vi "core.vi"(8 "H[5] in":u32[](array[numeric]), 11 "W[80]":u32[](array[numeric])) -> (0 "H[5] out":u32[](array[numeric]))   [LabVIEW 2013, in "SHA-1.lvlib" / "SHA-1.lvclass"]
uses:
  SHA-1.lvclass
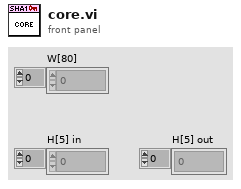
[diagram p1: front panel]
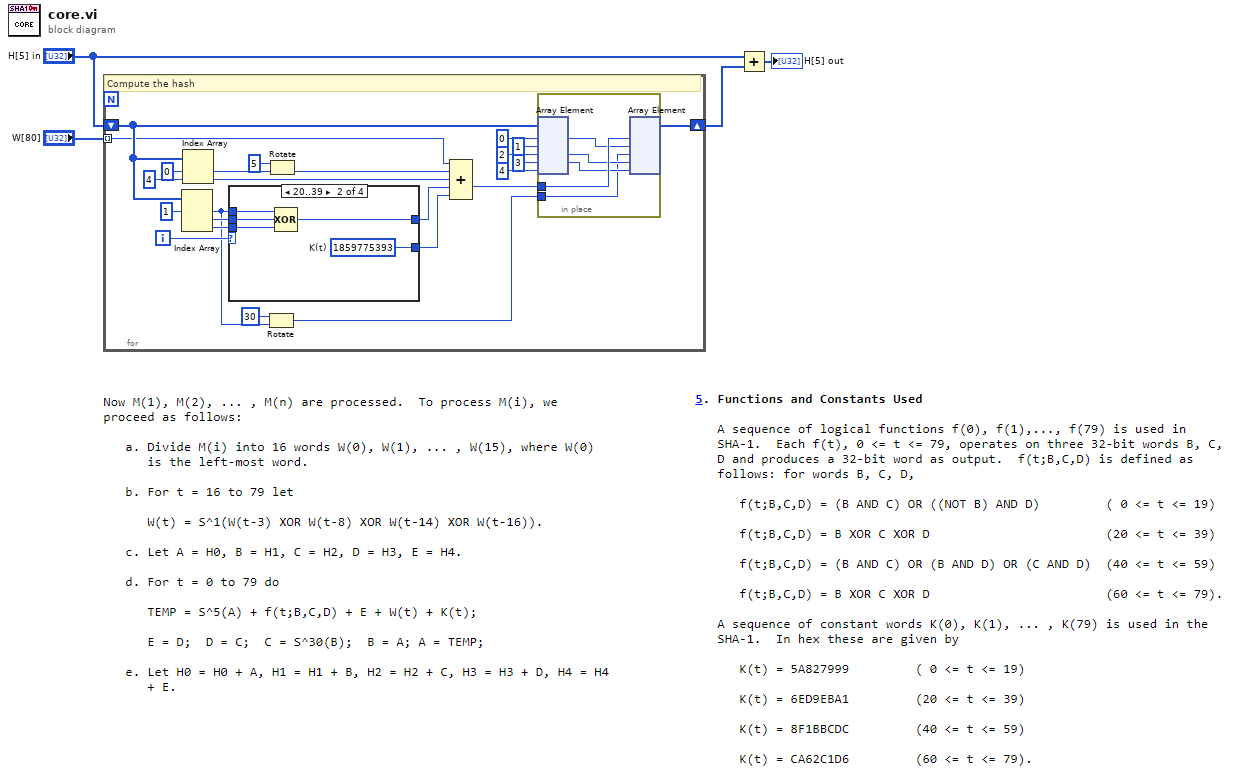
[diagram p0: block diagram]
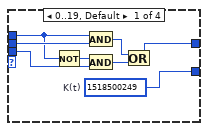
[diagram p2: hidden frame]
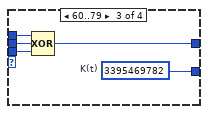
[diagram p3: hidden frame]
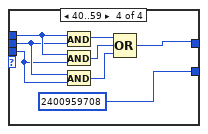
[diagram p4: hidden frame]
diagram:
  n1 = for {
    shift-right: [w9] -> w1
    shift-left: "H[5] in" -> [w18]
    tunnel: "W[80]" -> [w5] mode=indexing
    i -> [w28]
    # "Compute the hash"
    n2 = Index Array(array=w18, index #1=1 ("index")) -> (element #1=w16:u32, element #2=w21:u32, element #3=w20:u32)  [unwired: 2 in]
    n3 = Index Array(array=w18, index #1=0 ("index"), index #2=4 ("index")) -> (element #1=w24:u32, element #2=w7:u32)
    n4 = case shown="20..39" w28 {
      tunnel: w16 -> [w36 w46 w51 w59]
      tunnel: w21 -> [w37 w45 w50 w58]
      tunnel: w20 -> [w38 w44 w49 w57]
      tunnel: [w35 w42 w47 w53] -> w6
      tunnel: [w34 w43 w48 u32 2400959708] -> w8
      frame 0..19, Default {
        w34 = u32 1518500249  # K(t)
        n5 = Not(x=w36) -> (.not. x?=w41:u32)
        n6 = And(x=w36, y=w37) -> (x .and. y?=w39:u32)
        n7 = And(x=w41, y=w38) -> (x .and. y?=w40:u32)
        n8 = Or(x=w39, y=w40) -> (x .or. y?=w35:u32)
      }
      frame 20..39 {
        w43 = u32 1859775393  # K(t)
        n9 = Compound Arithmetic op=XOR(w46, w45, w44) -> (w42:u32)
      }
      frame 60..79 {
        w48 = u32 3395469782  # K(t)
        n10 = Compound Arithmetic op=XOR(w51, w50, w49) -> (w47:u32)
      }
      frame 40..59 {
        n11 = And(x=w59, y=w58) -> (x .and. y?=w56:u32)
        n12 = And(x=w59, y=w57) -> (x .and. y?=w55:u32)
        n13 = And(x=w58, y=w57) -> (x .and. y?=w54:u32)
        n14 = Compound Arithmetic op=OR(w56, w55, w54) -> (w53:u32)
      }
    }
    n15 = Rotate(1:w16, 2:i8 30 ("y")) -> (0:w10:u32)
    n16 = Rotate(1:w24, 2:i8 5 ("y")) -> (0:w23:u32)
    n17 = Compound Arithmetic op=ADD(w5, w23, w7, w6, w8) -> (w19:u32)
    n18 = in-place {
      in-place-border: w19 -> [w33]
      in-place-border: w10 -> [w29]
      n19 = in-place-array #1(w18, 0, 1, 2, 3, 4) -> (w32:u32, w31:u32, w30:u32)  [unwired: 2 out]
      n20 = in-place-array #1(w33, w32, w29, w31, w30) -> (w9:u32[])  [unwired: 5 out]
    }
  }
  n21 = Add(x="H[5] in", y=w1) -> (x+y=→"H[5] out":u32[])
